vi "generate_config_2Chann_simultaneous.vi"(4 "new task name":string, 5 "Generate config Chann2":T1={"maximum value"=5.0, "minimum value"=-5.0, "phase"=180.0, "amplitude"=1.0, "frequency"=10.0, "Wave Type"=0, "offset"=0.0} {"offset" format="%0.2p"; "Wave Type" items=["Sine", "Square", "Triangle", "Sawtooth", "DC Signal"]; "frequency" format="%0.2p"; "amplitude" format="%0.2p"}, 6 "Analog Out Channels":cluster{"0":bool, "1":bool}={"0"=TRUE, "1"=TRUE}, 7 "Generate config Chann1":T1={"maximum value"=5.0, "minimum value"=-5.0, "phase"=180.0, "amplitude"=1.0, "frequency"=10.0, "Wave Type"=0, "offset"=0.0} {"offset" format="%0.2p"; "Wave Type" items=["Sine", "Square", "Triangle", "Sawtooth", "DC Signal"]; "frequency" format="%0.2p"; "amplitude" format="%0.2p"}) -> (0 "error out":errorcluster, 1 "real frequency(Hz)":dbl, 2 "signal Generated":waveform(dbl)[](graph), 3 "task out":refnum<k21>)   [LabVIEW 2017]
uses:
  <vilib>/DAQmx/write.llb/DAQmx Write (Analog 1D Wfm NChan NSamp).vi
  <vilib>/DAQmx/create/channels.llb/DAQmx Create Channel (AO-Voltage-Basic).vi
  <vilib>/DAQmx/configure/timing.llb/DAQmx Timing (Use Waveform).vi
  <vilib>/Waveform/WDTOps.llb/WDT Append Waveforms DBL.vi
  <vilib>/DAQmx/miscellaneous.llb/DAQmx Fill In Error Info.vi
  <instrlib>/NI USB-6356/NI USB-6356.lvlib
  <vilib>/gmath/NI_Gmath.lvlib
panel:
  out "x-y*floor(x/y) 2":dbl
  out "x-y*floor(x/y)":dbl
  out "appended array 2":dbl[](array[numeric])
  out "appended array":dbl[](array[numeric])
  out "Y 2":dbl[](array[numeric])
  out "Y":dbl[](array[numeric])
  out "size(s) 2":i32
  out "size(s)":i32
  out "lcm":dbl
  out "cycles chann2":i32
  out "cycles chann1":i32
  out "real frequency(Hz) 2":dbl
  in  "error in":errorcluster
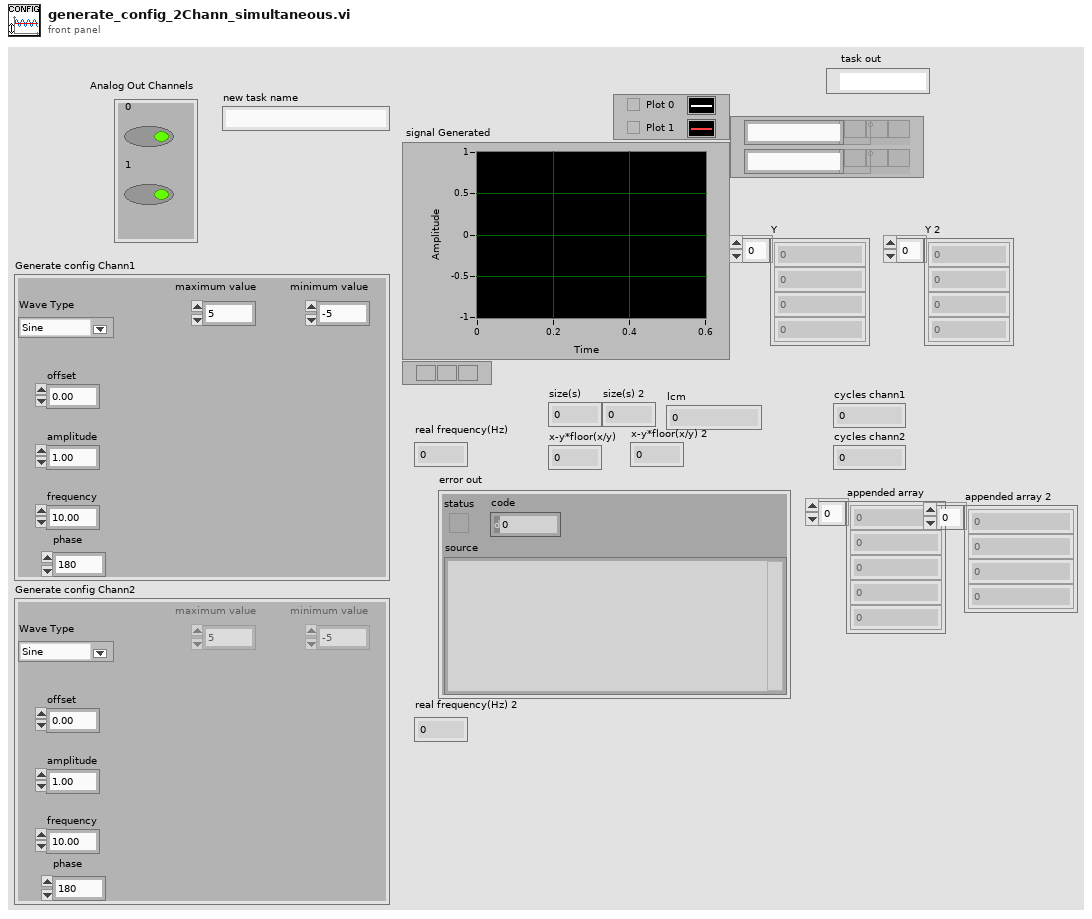
[diagram p1: front panel]
types:
  T1 = cluster{"maximum value":dbl, "minimum value":dbl, "phase":dbl, "amplitude":dbl, "frequency":dbl, "Wave Type":u16, "offset":dbl}
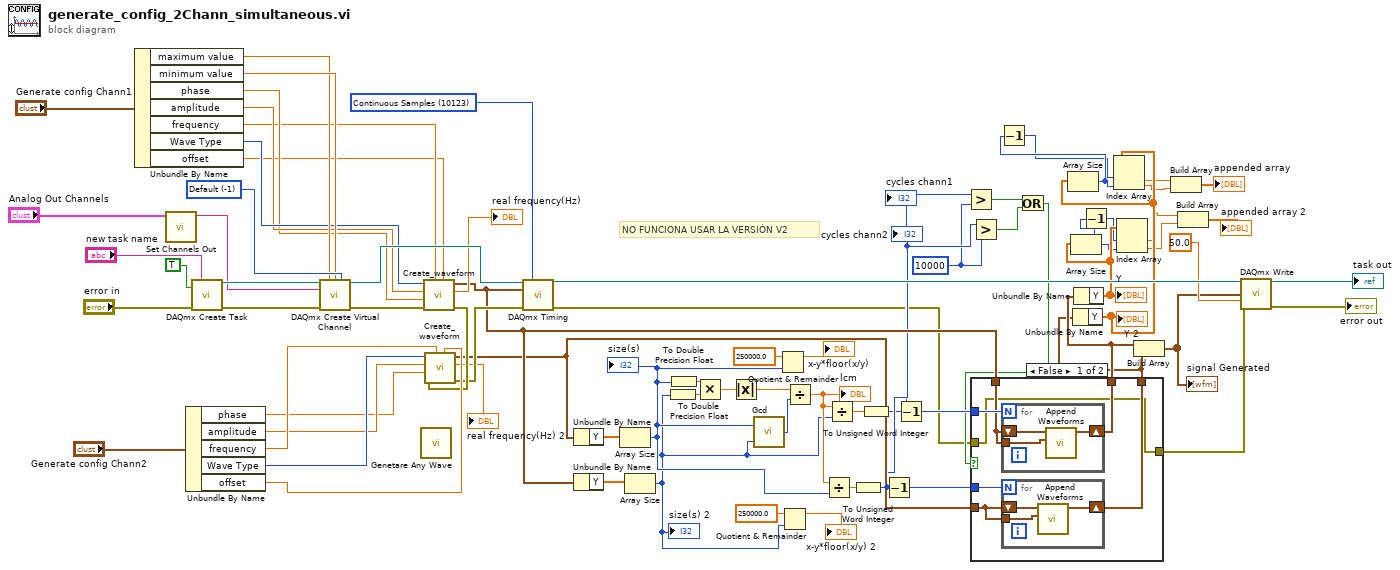
[diagram p0: block diagram]
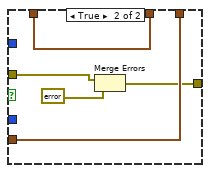
[diagram p2: hidden frame]
diagram:
  w27 = 10000
  w72 = 10123 items=["Finite Samples"=10178, "Continuous Samples"=10123, "Hardware Timed Single Point"=12522] ("sample mode")
  w76 = -1 items=["Default"=-1, "RSE"=10083, "Differential"=10106, "Pseudodifferential"=12529] ("output terminal configuration")
  # "NO FUNCIONA USAR LA VERSIÓN V2"
  n1 = Unbundle By Name("Generate config Chann1") -> ("maximum value"=w60:dbl, "minimum value"=w61:dbl, "phase"=w57:dbl, "amplitude"=w58:dbl, "frequency"=w56:dbl, "Wave Type"=w59:u16, "offset"=w55:dbl)
  n2 = call <instrlib>:"Set Channels Out.vi"("Analog Out Channels"="Analog Out Channels") -> ("String"=w36:string)  [unwired: 10 in]
  n3 = Unbundle By Name("Generate config Chann2") -> ("phase"=w49:dbl, "amplitude"=w50:dbl, "frequency"=w53:dbl, "Wave Type"=w51:u16, "offset"=w52:dbl)
  n4 = call <vilib>:"DAQmx Create Task.vi"("new task name"="new task name", "auto cleanup"=TRUE, "error in"="error in") -> ("task out"=w66:refnum<k21>, "error out"=w65:errorcluster)  [unwired: 11 in]
  n5 = call-poly <vilib>:"DAQmx Create Virtual Channel.vi"("task in"=w66, "maximum value"=w60, "minimum value"=w61, "output terminal configuration"=w76, "physical channels"=w36, "error in"=w65) -> ("task out"=w75:refnum<k21>, "error out"=w74:errorcluster)  [unwired: 8 in]
  n6 = call <instrlib>:"Genetare Any Wave.vi"() -> ()  [unwired: 18 in, 2 out]
  n7 = call "Create_waveform.vi"("offset"=w55, "frequency"=w56, "error in"=w74, "phase"=w57, "amplitude"=w58, "Wave Type"=w59) -> ("error out"=w48:errorcluster, "real frequency(Hz)"=→"real frequency(Hz)":dbl, "signal Generated"=w32:waveform(dbl))  [unwired: 3 in]
  n8 = call "Create_waveform.vi"("offset"=w52, "frequency"=w53, "error in"=w48, "phase"=w49, "amplitude"=w50, "Wave Type"=w51) -> ("error out"=w47:errorcluster, "real frequency(Hz)"=→"real frequency(Hz) 2":dbl, "signal Generated"=w31:waveform(dbl))  [unwired: 3 in]
  n9 = call-poly <vilib>:"DAQmx Timing.vi"("task/channels in"=w75, "sample mode"=w72, "waveform"=w32, "error in"=w47) -> ("task out"=w73:refnum<k21>, "error out"=w22:errorcluster)  [unwired: 10 in]
  n10 = Unbundle By Name(w31) -> ("Y"=w44:dbl[])
  n11 = Unbundle By Name(w32) -> ("Y"=w43:dbl[])
  n12 = Array Size(array=w44) -> (size(s)=w5:i32)
  "size(s)" <- w5
  n13 = Array Size(array=w43) -> (size(s)=w3:i32)
  "size(s) 2" <- w3
  n14 = To Double Precision Float(number=w3) -> (double precision float=w35:dbl)
  n15 = To Double Precision Float(number=w5) -> (double precision float=w34:dbl)
  n16 = Multiply(x=w34, y=w35) -> (x*y=w33:dbl)
  n17 = Absolute Value(x=w33) -> (abs(x)=w42:dbl)
  n18 = call <vilib>:"Gcd.vi"("y"=w3, "x"=w5) -> ("gcd(x,y)"=w41:i32)
  n19 = Quotient & Remainder(x=250000.0, y=w5) -> (x-y*floor(x/y)=→"x-y*floor(x/y)":dbl)  [unwired: 1 out]
  n20 = Quotient & Remainder(x=250000.0, y=w3) -> (x-y*floor(x/y)=→"x-y*floor(x/y) 2":dbl)  [unwired: 1 out]
  n21 = Divide(x=w42, y=w41) -> (x/y=w40:dbl)
  "lcm" <- w40
  n22 = Divide(x=w40, y=w5) -> (x/y=w29:dbl)
  n23 = Divide(x=w40, y=w3) -> (x/y=w39:dbl)
  n24 = To Unsigned Word Integer(number=w29) -> (unsigned 16bit integer=w28:u16)
  "cycles chann2" <- w28
  n25 = To Unsigned Word Integer(number=w39) -> (unsigned 16bit integer=w26:u16)
  "cycles chann1" <- w26
  n26 = Decrement(x=w28) -> (x-1=w37:u16)
  n27 = Decrement(x=w26) -> (x-1=w38:u16)
  n28 = Greater?(x=w26, y=w27) -> (0:w25:bool)
  n29 = Greater?(x=w28, y=w27) -> (0:w24:bool)
  n30 = Or(x=w25, y=w24) -> (x .or. y?=w23:bool)
  n31 = case shown="False" w23 {
    tunnel: [w83 w94] -> w20
    tunnel: [w82 w93] -> w19
    tunnel: w38 -> [w81 _]
    tunnel: w37 -> [w80 _]
    tunnel: w32 -> [w79 w94]
    tunnel: w31 -> [w78 w93]
    tunnel: w22 -> [w77 w92]
    tunnel: [w77 w91] -> w21
    frame False {
      n32 = for {
        N: w81 -> [_]
        shift-right: [w87] -> w83
        shift-left: w79 -> [w89]
        tunnel: w79 -> [w88]
        n33 = call-poly <vilib>:"Append Waveforms.vi"("waveform B"=w88, "waveform A"=w89) -> ("waveform out"=w87:waveform(dbl))  [unwired: 8 in, 1 out]
      }
      n34 = for {
        N: w80 -> [_]
        shift-right: [w84] -> w82
        shift-left: w78 -> [w86]
        tunnel: w78 -> [w85]
        n35 = call-poly <vilib>:"Append Waveforms.vi"("waveform B"=w85, "waveform A"=w86) -> ("waveform out"=w84:waveform(dbl))  [unwired: 8 in, 1 out]
      }
    }
    frame True {
      n36 = Merge Errors(w92, errorcluster {"status"=TRUE, "code"=0, "source"="Change frequencies to\nbe multiple between them"} ("error IO")) -> (w91:errorcluster)
    }
  }
  n37 = Unbundle By Name(w19) -> ("Y"=w17:dbl[])
  "Y 2" <- w17
  n38 = Array Size(array=w17) -> (size(s)=w15:i32)
  n39 = Decrement(x=w15) -> (x-1=w14:i32)
  n40 = Unbundle By Name(w20) -> ("Y"=w18:dbl[])
  "Y" <- w18
  n41 = Array Size(array=w18) -> (size(s)=w10:i32)
  n42 = Decrement(x=w10) -> (x-1=w16:i32)
  n43 = Index Array(array=w17, index #1=w14, index #2=w15) -> (element #1=w13:dbl, element #2=w12:dbl)
  n44 = Index Array(array=w18, index #1=w16, index #2=w10) -> (element #1=w8:dbl, element #2=w9:dbl)
  n45 = Build Array(w20, w19) -> (w30:waveform(dbl)[])
  "signal Generated" <- w30
  n46 = Build Array(w13, w12) -> (→"appended array":dbl[])
  n47 = Build Array(w8, w9) -> (→"appended array 2":dbl[])
  n48 = call-poly <vilib>:"DAQmx Write.vi"("task/channels in"=w73, "data"=w30, "timeout"=50.0, "error in"=w21) -> ("task out"=→"task out":refnum<k21>, "error out"=→"error out":errorcluster)  [unwired: 9 in, 1 out]
